vi "Word_Update_Chart.vi"(0 "Word.InlineShapes":refnum<k7>, 1 "chart data":dbl[][](array[numeric]) format="%.2f", 9 "Chart index":u16, 11 "error in":errorcluster, 12 "column header":string[](array[string]), 13 "row header":string[](array[string])) -> (15 "error out":errorcluster)   [LabVIEW 2017, in "NI_ReportGenerationToolkit.lvlib"]
uses:
  <vilib>/addons/_office/NI_ReportGenerationToolkit.lvlib
panel:
  in  "MS Graph":refnum<k7>
  in  "Graph.Chart":refnum<k7>
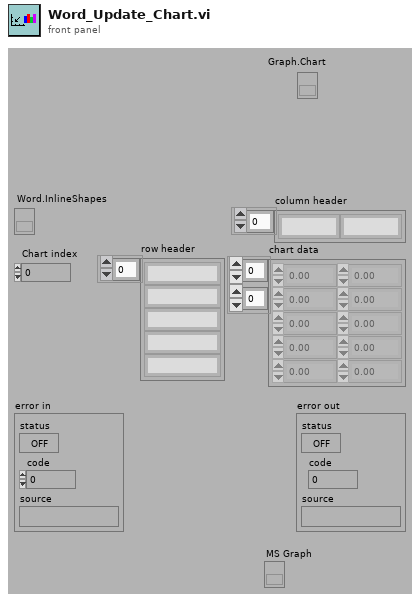
[diagram p1: front panel]
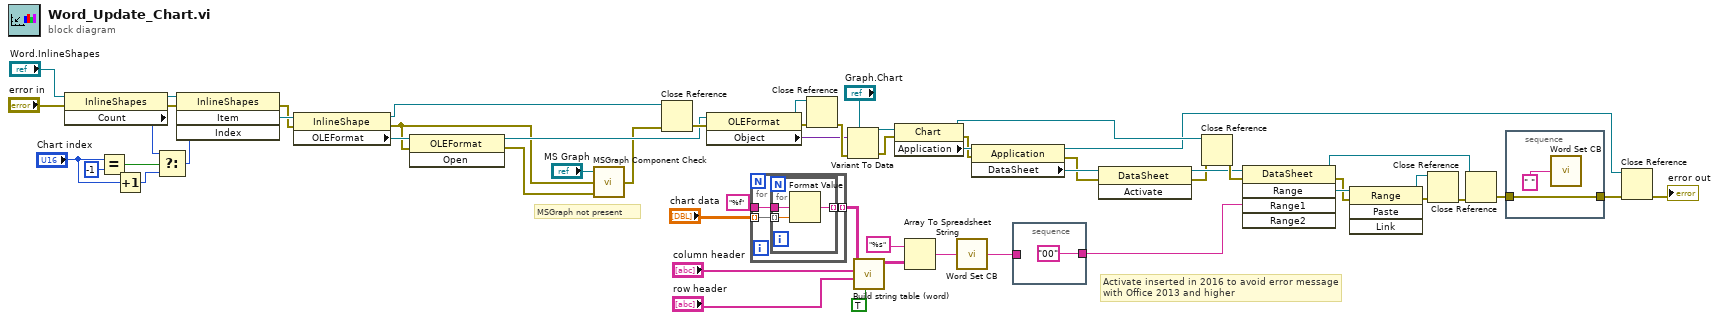
[diagram p0: block diagram]
diagram:
  # "Activate inserted in 2016 to avoid error message \nwith Office 2013 and higher"
  # "MSGraph not present"
  n1 = property class="InlineShapes"(reference="Word.InlineShapes", error in="error in") -> (reference out=w44:refnum<k7>, error out=w49:errorcluster, "Count"=w36:i32)
  n2 = Equal?(x="Chart index", y=i16 -1) -> (x = y?=w43:bool)
  n3 = Increment(x="Chart index") -> (x+1=w41:u16)
  n4 = Select(t=w36, s=w43, f=w41) -> (s? t:f=w40:i32)
  n5 = invoke class="InlineShapes" method="Item"(reference=w44, error in=w49, "Index"=w40) -> (error out=w45:errorcluster, "Item"=w46:refnum<k7>)  [unwired: 1 in, 2 out]
  n6 = property class="InlineShape"(reference=w46, error in=w45) -> (reference out=w48:refnum<k7>, error out=w8:errorcluster, "OLEFormat"=w13:refnum<k7>)
  n7 = invoke class="OLEFormat" method="Open"(reference=w13, error in=w8) -> (reference out=w12:refnum<k7>, error out=w7:errorcluster)  [unwired: 1 in, 1 out]
  n8 = call <vilib>:"MSGraph Component Check.vi"("error 2"=w7, "error 1"=w8, "MS Graph"="MS Graph") -> ("error out"=w6:errorcluster)
  n9 = Close Reference(reference=w48, error in (no error)=w6) -> (error out=w47:errorcluster)
  n10 = property class="OLEFormat"(reference=w12, error in=w47) -> (reference out=w33:refnum<k7>, error out=w34:errorcluster, "Object"=w35:variant)
  n11 = for {
    tunnel: "chart data" -> [w59] mode=indexing
    tunnel: "%f" -> [w58]
    tunnel: [w57] -> w32 mode=indexing
    n12 = for {
      tunnel: w59 -> [w62] mode=indexing
      tunnel: w58 -> [w61]
      tunnel: [w60] -> w57 mode=indexing
      n13 = Format Value(format string=w61, value (0)=w62) -> (output string=w60:string)  [unwired: 1 out]
    }
  }
  n14 = Close Reference(reference=w33, error in (no error)=w34) -> (error out=w51:errorcluster)
  n15 = Variant To Data(error in=w51, type="Graph.Chart", Variant=w35) -> (data=w55:refnum<k7>, error out=w50:errorcluster)
  n16 = call <vilib>:"Build string table (word).vi"("Graph data?"=TRUE, "row headers"="row header", "column headers"="column header", "text data"=w32) -> ("output table"=w30:string[][])  [unwired: 7 out]
  n17 = property class="Chart"(reference=w55, error in=w50) -> (reference out=w52:refnum<k7>, error out=w53:errorcluster, "Application"=w54:refnum<k7>)
  n18 = Array To Spreadsheet String(array=w30, 3:"%s" ("format string")) -> (spreadsheet string=w11:string)  [unwired: 1 out]
  n19 = call <vilib>:"Word Set CB.vi"("String"=w11) -> ("String 2"=w10:string)
  n20 = property class="Application"(reference=w54, error in=w53) -> (reference out=w15:refnum<k7>, error out=w2:errorcluster, "DataSheet"=w4:refnum<k7>)
  n21 = stacked-sequence {
    tunnel: ["00"] -> w17
    tunnel: w10 -> [_]
    frame #0 {
    }
  }
  n22 = invoke class="DataSheet" method="Activate"(reference=w4, error in=w2) -> (reference out=w3:refnum<k7>, error out=w1:errorcluster)  [unwired: 1 in, 1 out]
  n23 = Close Reference(reference=w52, error in (no error)=w1) -> (error out=w20:errorcluster)
  n24 = invoke class="DataSheet" method="Range"(reference=w3, error in=w20, "Range1"=w17) -> (reference out=w22:refnum<k7>, error out=w21:errorcluster, "Range"=w23:refnum<k7>)  [unwired: 2 in, 2 out]
  n25 = invoke class="Range" method="Paste"(reference=w23, error in=w21) -> (reference out=w25:refnum<k7>, error out=w26:errorcluster)  [unwired: 2 in, 2 out]
  n26 = Close Reference(reference=w25, error in (no error)=w26) -> (error out=w24:errorcluster)
  n27 = Close Reference(reference=w22, error in (no error)=w24) -> (error out=w19:errorcluster)
  n28 = stacked-sequence {
    tunnel: w19 -> [w65]
    tunnel: [w65] -> w16
    frame #0 {
      n29 = call <vilib>:"Word Set CB.vi"("String"=" ") -> ()  [unwired: 1 out]
    }
  }
  n30 = Close Reference(reference=w15, error in (no error)=w16) -> (error out=→"error out":errorcluster)
